vi "One Session One Pin Group One Instrument One Site - DCPower.vi"(8 "error in":errorcluster) -> (0 "error out":errorcluster, 3 "session reservation out":refnum<class "Session Reservation.lvclass">)   [LabVIEW 2020, in "MeasurementServerTests.lvlib"]
uses:
  MeasurementServerTests.lvlib
  Runtime/MeasurementLink Session Management V1/Session Reservation/Session Reservation.lvclass
  TestUtilities/TestUtilities.Runtime/Session Reservation Test Utilities/Session Reservation Test Utilities.lvlib
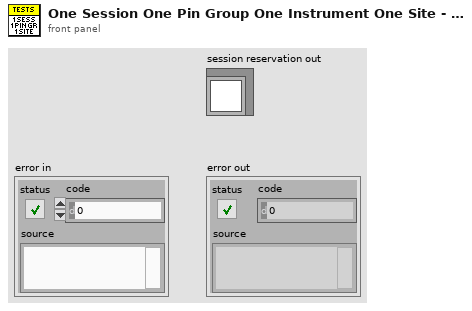
[diagram p1: front panel]
types:
  T1 = typedef "MeasurementLink Session Management V1.lvlib/Session Reservation.lvclass/Data.ctl" = cluster{"session and driver infos":T2[], "pin or relay names":string[], "connection map":refnum<class "Connection Map.lvclass">, "pin map context":T7, "reservation observer":refnum<class "IReservation Observer.lvclass">, "dvr valid":bool, "group mappings":T8}
  T2 = typedef "MeasurementLink Session Management V1.lvlib/Session Reservation.lvclass/Session and Driver Info.ctl" = cluster{"session info":T3, "session":variant, "session factory":refnum<class "ISession Factory.lvclass">, "initialize and close session behavior":T6}
  T3 = typedef "MeasurementLink Session Management Client.lvlib/ni_measurementlink_sessionmanagement_v1_SessionInformation.ctl" = cluster{"session":T4, "resource_name":string, "channel_list":string, "instrument_type_id":string, "session_exists":bool, "channel_mappings":T5[]}
  T4 = typedef "MeasurementLink Session Management Client.lvlib/nidevice_grpc_Session.ctl" = cluster{"name":string}
  T5 = typedef "MeasurementLink Session Management Client.lvlib/ni_measurementlink_sessionmanagement_v1_ChannelMapping.ctl" = cluster{"pin_or_relay_name":string, "site":i32, "channel":string, "multiplexer_resource_name":string, "multiplexer_route":string}
  T6 = typedef "MeasurementLink Instrument.lvlib/ISession Factory.lvclass/Initialize and Close Session Behavior.ctl" = enum16{"Initialize and Close", "Attach and Detach", "Initialize and Detach", "Attach and Close"}
  T7 = typedef "MeasurementLink Session Management Client.lvlib/ni_measurementlink_PinMapContext.ctl" = cluster{"pin_map_id":string, "sites":i32[]}
  T8 = typedef "MeasurementLink Session Management V1.lvlib/Session Reservation.lvclass/Group Mapping.ctl" = map{string, string[]}
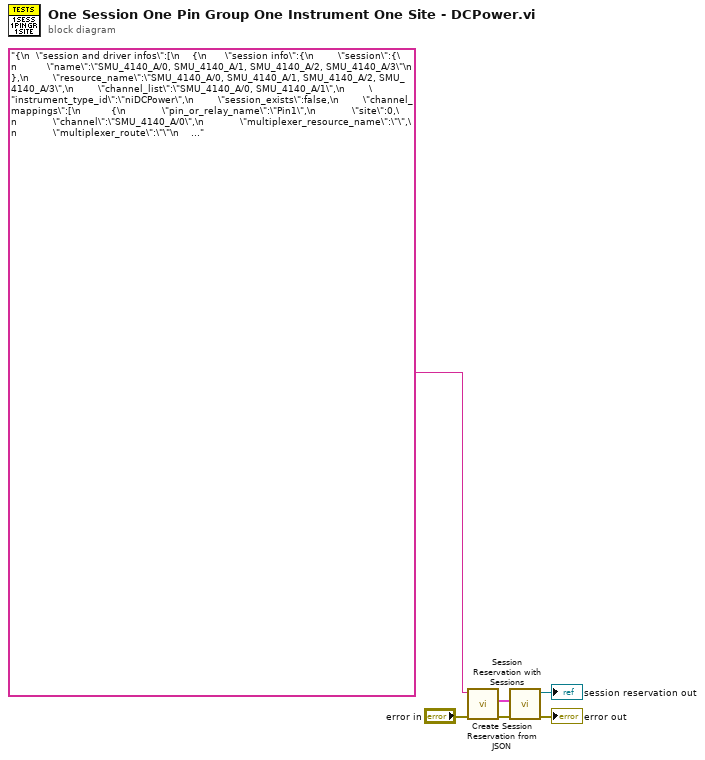
[diagram p0: block diagram]
diagram:
  n1 = call "Create Session Reservation from JSON.vi"("error in"="error in", "json"="{\n  \"session and driver infos\":[\n    {\n      \"session info\":{\n        \"session\":{\n          \"name\":\"SMU_4140_A/0, SMU_4140_A/1, SMU_4140_A/2, SMU_4140_A/3\"\n        },\n        \"resource_name\":\"SMU_4140_A/0, SMU_4140_A/1, SMU_4140_A/2, SMU_4140_A/3\",\n        \"channel_list\":\"SMU_4140_A/0, SMU_4140_A/1\",\n        \"instrument_type_id\":\"niDCPower\",\n        \"session_exists\":false,\n        \"channel_mappings\":[\n          {\n            \"pin_or_relay_name\":\"Pin1\",\n            \"site\":0,\n            \"channel\":\"SMU_4140_A/0\",\n            \"multiplexer_resource_name\":\"\",\n            \"multiplexer_route\":\"\"\n          },\n          {\n            \"pin_or_relay_name\":\"Pin2\",\n            \"site\":0,\n            \"channel\":\"SMU_4140_A/1\",\n            \"multiplexer_resource_name\":\"\",\n            \"multiplexer_route\":\"\"\n          }\n        ]\n      },\n      \"\":null,\n      \"session factory\":\"§§AAAAATsgTWVhc3VyZW1lbnRMaW5rIEluc3RydW1lbnQubHZsaWIYSVNlc3Npb24gRmFjdG9yeS5sdmNsYXNzAAAAAAAAAAAA\",\n      \"initialize and close session behavior\":\"Initialize and Close\"\n    }\n  ],\n  \"pin or relay names\":[\"PinGroup1\"],\n  \"connection map\":\"§§AAAAAUQrTWVhc3VyZW1lbnRMaW5rIFNlc3Npb24gTWFuYWdlbWVudCBWMS5sdmxpYhZDb25uZWN0aW9uIE1hcC5sdmNsYXNzAAAAAAABAAAAAAAAAAABBAAAAAEAAAAJbmlEQ1Bvd2VyAAAAAgAAAAEAAAACAAAABFBpbkEAAAAEUGluQQAAAAEAAAAJbmlEQ1Bvd2VyAAAAATEgAIAAAAAAAQAEAAAAAQAAAAAAAAAAAARQaW5CAAAABFBpbkIAAAABAAAACW5pRENQb3dlcgAAAAEyIACAAAAAAAEABAAAAAEAAAAAAAAAAAACAAAAAQAAAARQaW5BAAAABFBpbkEAAAACAAAACW5pRENQb3dlcgAAAAEzIACAAAAAAAEABAAAAAEAAAAAAAAAAAABAAAACW5pRENQb3dlcgAAAAIAAAABAAAAAgAAAAIAAAAEUGluQQAAAARQaW5C\",\n  \"pin map context\":{\n    \"pin_map_id\":\"PinGroupSupport\",\n    \"sites\":[0,1,2]\n  },\n  \"reservation observer\":\"§§AAAAAUsrTWVhc3VyZW1lbnRMaW5rIFNlc3Npb24gTWFuYWdlbWVudCBWMS5sdmxpYh1JUmVzZXJ2YXRpb24gT2JzZXJ2ZXIubHZjbGFzcwAAAAAAAAAAAA\",\n  \"dvr valid\":true,\n  \"group mappings\":[[\"PinGroup1\",[\"Pin1\",\"Pin2\"]]]\n}") -> ("error out"=w6:errorcluster, "data out"=w5:T1)  [unwired: 7 in, 1 out]
  n2 = call "Session Reservation with Sessions.vi"("error in"=w6, "data in"=w5) -> ("error out"=→"error out":errorcluster, "session reservation out"=→"session reservation out":refnum<class "Session Reservation.lvclass">)  [unwired: 7 in, 1 out]
